vi "MGCC_DataLog_global.vi"() -> ()   [LabVIEW 2016]
panel:
  in  "Sampling step":dbl
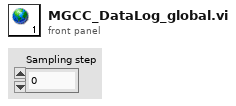
[diagram p1: front panel]
diagram:
